vi "Dialog Tester - Outputs.vi"() -> ()   [LabVIEW 2019]
doc: "<b>TEST VI</b> will check that the output values for pop ups with some type of output are passed correctly"
uses:
  Graphics.ctl
  Standard/Input (DBL)/Input (DBL).lvclass
  Pop-Up.lvlib
  Standard/Input (I32)/Input (I32).lvclass
  Standard/Input (String)/Input (String).lvclass
  Standard/Timeout Two Button/Timeout Two Button.lvclass
  Standard/Two Button/Two Button.lvclass
  Theme/Theme.lvclass
panel:
  out "Timeout":bool
  out "password":string
  out "Two-Button T.O. Choice?":bool
  out "Two-Button Choice?":bool
  out "Input Value (String)":string
  out "Input Value (I32)":i32
  out "Input Value (DBL)":dbl
  out "iteration":i32
  in  "Error In":errorcluster
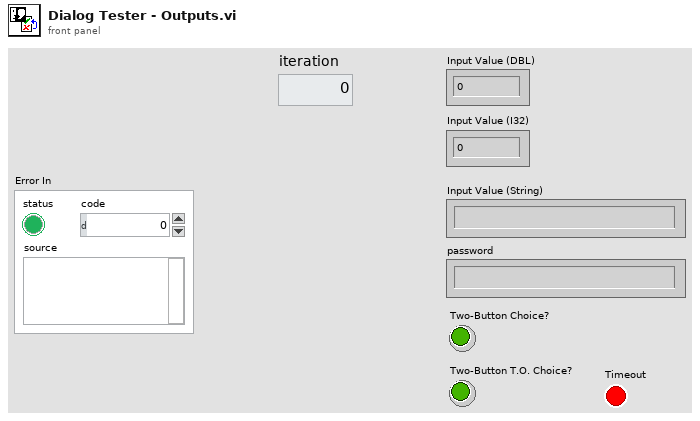
[diagram p1: front panel]
types:
  T1 = typedef "Pop-Up.lvlib/Graphics.ctl" = string
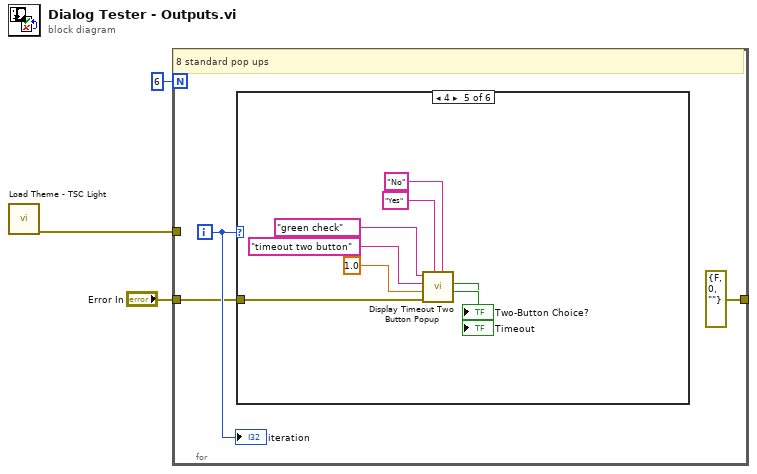
[diagram p0: block diagram]
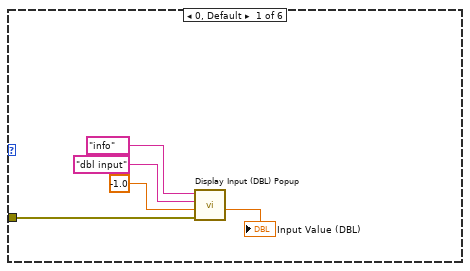
[diagram p2: hidden frame]
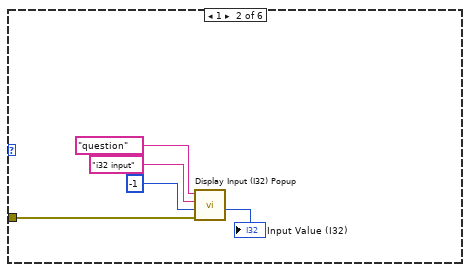
[diagram p3: hidden frame]
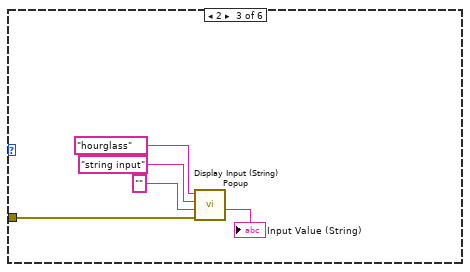
[diagram p4: hidden frame]
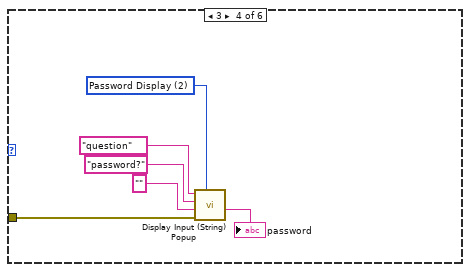
[diagram p5: hidden frame]
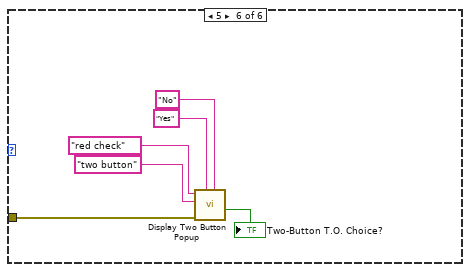
[diagram p6: hidden frame]
diagram:
  n1 = call "Load Theme - TSC Light.vi"() -> ("error out"=w1:errorcluster)  [unwired: 10 in, 1 out]
  n2 = for {
    N: 6 -> [_]
    tunnel: "Error In" -> [w5]
    tunnel: [errorcluster {"status"=FALSE, "code"=0, "source"=""} ("error constant")] -> _
    tunnel: w1 -> [_]
    i -> [w6]
    # "8 standard pop ups"
    n3 = case shown="4" w6 {
      tunnel: w5 -> [w11 w16 w21 w27 w35 w41]
      frame 0, Default {
        n4 = call "Display Input (DBL) Popup.vi"("error in"=w11, "Default Input"=-1.0, "Message"="dbl input", "Graphic"=T1 "info") -> ("Input Value"=→"Input Value (DBL)":dbl)  [unwired: 6 in, 1 out]
      }
      frame 1 {
        n5 = call "Display Input (I32) Popup.vi"("error in"=w16, "Default Input"=-1, "Message"="i32 input", "Graphic"=T1 "question") -> ("Input Value"=→"Input Value (I32)":i32)  [unwired: 6 in, 1 out]
      }
      frame 2 {
        n6 = call "Display Input (String) Popup.vi"("error in"=w21, "Default Input"="", "Message"="string input", "Graphic"=T1 "hourglass") -> ("Input Value"=→"Input Value (String)":string)  [unwired: 6 in, 1 out]
      }
      frame 3 {
        w22 = u32 2 items=["Normal Display", "'\\' Codes Display", "Password Display", "Hex Display"] ("Display Style")
        n7 = call "Display Input (String) Popup.vi"("Display Style"=w22, "error in"=w27, "Default Input"="", "Message"="password?", "Graphic"=T1 "question") -> ("Input Value"=→"password":string)  [unwired: 5 in, 1 out]
      }
      frame 4 {
        n8 = call "Display Timeout Two Button Popup.vi"("N-Text"="No", "Y-Text"="Yes", "error in"=w35, "Timeout (s)"=1.0 ("Default Input"), "Message"="timeout two button", "Graphic"=T1 "green check") -> ("Choice"=→"Two-Button Choice?":bool, "Timeout"=→"Timeout":bool)  [unwired: 3 in, 1 out]
      }
      frame 5 {
        n9 = call "Display Two Button Popup.vi"("N-Text"="No", "Y-Text"="Yes", "error in"=w41, "Message"="two button", "Graphic"=T1 "red check") -> ("Choice"=→"Two-Button T.O. Choice?":bool)  [unwired: 5 in, 1 out]
      }
    }
    "iteration" <- w6
  }
